vi "Goto.vi"(7 "Speed":i32, 8 "error in (no error)":errorcluster, 9 "Direction":enum16{""}(ring), 10 "New Position":enum16{""}(ring), 11 "TranslationStage in":refnum<class "ArduinoTranslationStage.lvclass">) -> (0 "error out":errorcluster, 3 "TranslationStage out":refnum<class "ArduinoTranslationStage.lvclass">)   [LabVIEW 2023, in "ArduinoTranslationStage.lvlib" / "ArduinoTranslationStage.lvclass"]
uses:
  ArduinoTranslationStage.lvclass
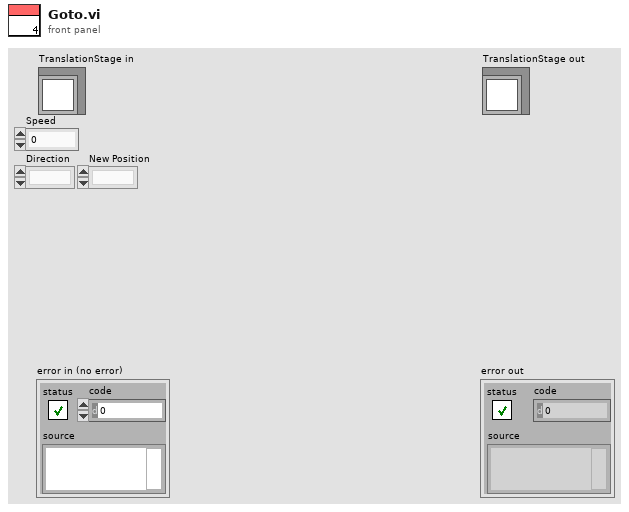
[diagram p1: front panel]
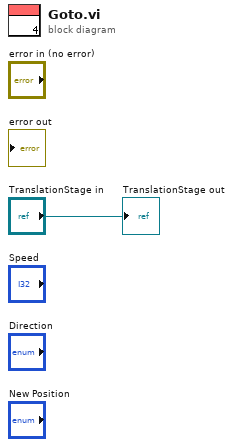
[diagram p0: block diagram]
diagram:
  "TranslationStage out" <- "TranslationStage in"
